vi "PXI-AO Gain Bank.vi"(0 "AO Channels":i32[](array[numeric]), 2 "Action":T1(ring), 5 "Gains":dbl[](array[numeric]), 7 "AO channel":i32, 11 "error in (no error)":errorcluster) -> (4 "Channels":i32[](array[numeric]), 6 "Gains out":dbl[](array[numeric]), 8 "Gains at setup":dbl[](array[numeric]), 10 "Gain Compensation Factors":dbl[](array[numeric]), 14 "Gain 1 channel":dbl, 15 "error out":errorcluster)   [LabVIEW 2020]
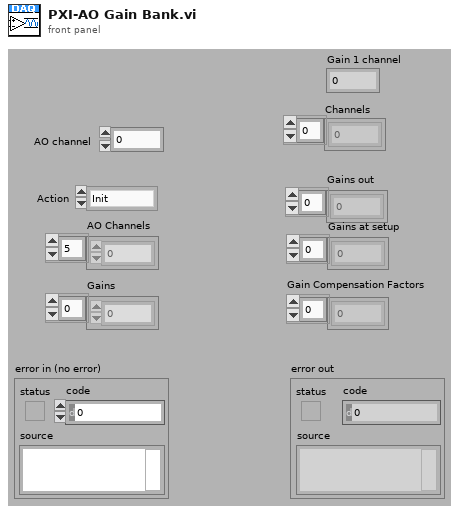
[diagram p1: front panel]
types:
  T1 = enum16{"Init", "Write", "Read", "Latch setup", "Compute comp.", "Read 1 Channel"}
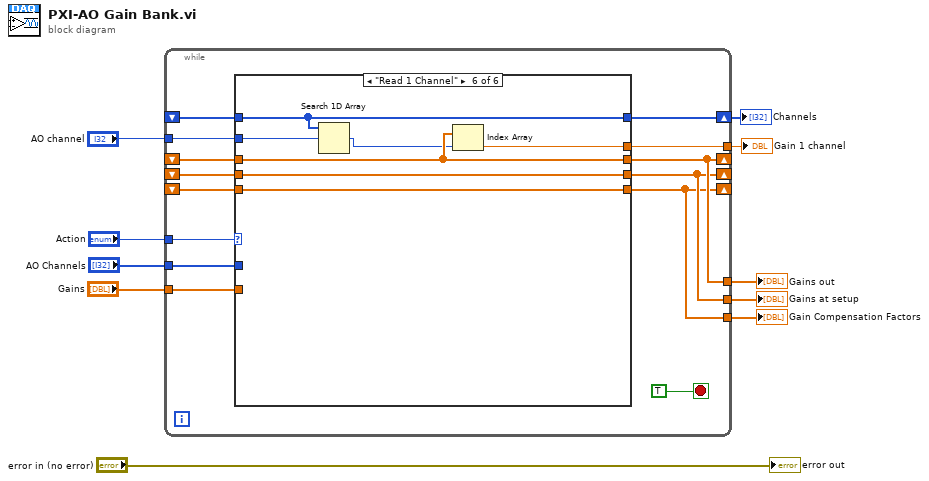
[diagram p0: block diagram]
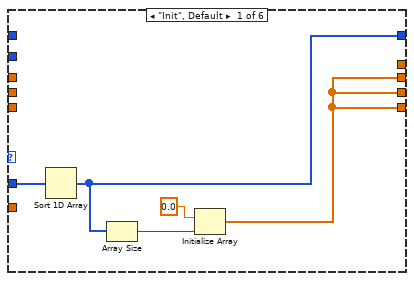
[diagram p2: hidden frame]
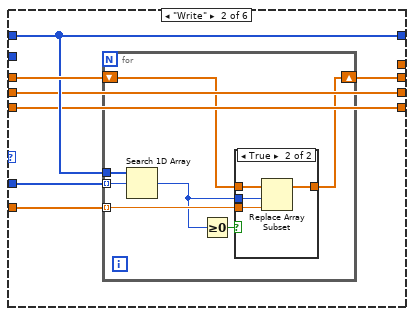
[diagram p3: hidden frame]
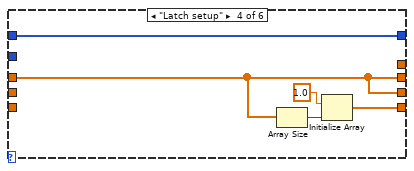
[diagram p6: hidden frame]
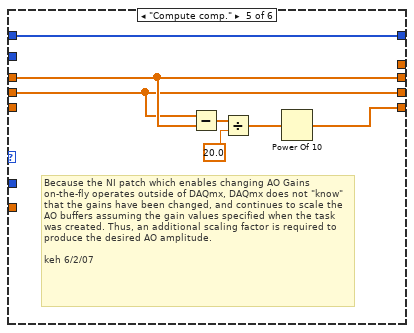
[diagram p7: hidden frame]
diagram:
  n1 = while {
    tunnel: "Action" -> [w23]
    tunnel: "AO Channels" -> [w22]
    shift-right: [w15] -> _
    shift-left: _ -> [w21]
    tunnel: "Gains" -> [w20]
    shift-right: [w19] -> w6
    shift-left: _ -> [w18]
    shift-right: [w14] -> _
    shift-left: _ -> [w17]
    shift-right: [w13] -> _
    shift-left: _ -> [w16]
    tunnel: [w15] -> w5
    tunnel: [w14] -> w4
    tunnel: [w13] -> w3
    tunnel: "AO channel" -> [w12]
    tunnel: [w11] -> w1
    stop <- TRUE stop-if-true
    n2 = case shown="\"Read 1 Channel\"" w23 {
      tunnel: w22 -> [w29 w36 _ _ _ _]
      tunnel: [w26 w30 w51 w54 w61 w67] -> w15
      tunnel: w21 -> [_ w35 w51 w54 w61 w67]
      tunnel: w20 -> [_ w34 _ _ _ _]
      tunnel: [w28 w33 w52 w55 w58 w69] -> w19
      tunnel: w18 -> [_ w33 w52 w55 w58 w69]
      tunnel: [w26 w32 w50 w54 w60 w70] -> w14
      tunnel: [w26 w31 w49 w53 w59 w71] -> w13
      tunnel: w17 -> [_ w32 w50 _ w60 w70]
      tunnel: w16 -> [_ w31 w49 _ _ w71]
      tunnel: w12 -> [_ _ _ _ _ w68]
      tunnel: [_ _ _ _ _ w65] -> w11
      frame "Init", Default {
        n3 = Sort 1D Array(array=w29) -> (sorted array=w28:i32[])
        n4 = Array Size(array=w28) -> (size(s)=w25:i32)
        n5 = Initialize Array(0.0 ("element"), w25) -> (w26:dbl[])
      }
      frame "Write" {
        n6 = for {
          tunnel: w36 -> [w39] mode=indexing
          tunnel: w34 -> [w42] mode=indexing
          tunnel: w33 -> [w40]
          shift-right: [w43] -> w30
          shift-left: w35 -> [w41]
          n7 = Search 1D Array(1D array=w40, element=w39) -> (index of element=w37:i32)  [unwired: 1 in]
          n8 = Greater Or Equal To 0?(x=w37) -> (x >= 0?=w38:bool)
          n9 = case shown="True" w38 {
            tunnel: w41 -> [w44 w48]
            tunnel: [w44 w47] -> w43
            tunnel: w37 -> [_ w46]
            tunnel: w42 -> [_ w45]
            frame False {
            }
            frame True {
              n10 = Replace Array Subset(array=w48, new element=w45, index=w46) -> (w47:dbl[])
            }
          }
        }
      }
      frame "Read" {
      }
      frame "Latch setup" {
        n11 = Array Size(array=w54) -> (size(s)=w57:i32)
        n12 = Initialize Array(1.0 ("element"), w57) -> (w53:dbl[])
      }
      frame "Compute comp." {
        # "Because the NI patch which enables changing AO Gains on-the-fly operates outside of DAQmx, DAQmx does not \"know\" that the gains have been changed, and continues to scale the AO buffers assuming the gain values specified when the task was created. Thus, an additional scaling factor is required to produce the desired AO amplitude.\n\nkeh 6/2/07"
        n13 = Subtract(x=w60, y=w61) -> (x-y=w64:dbl[])
        n14 = Divide(x=w64, y=20.0 ("Numeric")) -> (x/y=w62:dbl[])
        n15 = Power Of 10(x=w62) -> (10^x=w59:dbl[])
      }
      frame "Read 1 Channel" {
        n16 = Search 1D Array(1D array=w69, element=w68) -> (index of element=w66:i32)  [unwired: 1 in]
        n17 = Index Array(array=w67, index=w66) -> (element=w65:dbl)
      }
    }
  }
  "Gains out" <- w5
  "Gain Compensation Factors" <- w3
  "Gains at setup" <- w4
  "Channels" <- w6
  "Gain 1 channel" <- w1
  "error out" <- "error in (no error)"
